vi "PlotMotionProfile.vi"(1 "Trajectory Points":T3[](array[typedef]) {"Time (ms)" items=["TrajectoryDuration_0ms"=0, "TrajectoryDuration_5ms"=5, "TrajectoryDuration_10ms"=10, "TrajectoryDuration_20ms"=20, "TrajectoryDuration_30ms"=30, "TrajectoryDuration_40ms"=40, "TrajectoryDuration_50ms"=50, "TrajectoryDuration_100ms"=100]}) -> (0 "MotionProfileGraph":T2 {"Trajectory Point Interval (ms)" items=["TrajectoryDuration_0ms"=0, "TrajectoryDuration_5ms"=5, "TrajectoryDuration_10ms"=10, "TrajectoryDuration_20ms"=20, "TrajectoryDuration_30ms"=30, "TrajectoryDuration_40ms"=40, "TrajectoryDuration_50ms"=50, "TrajectoryDuration_100ms"=100]})   [LabVIEW 2018, in "ArgosLib.lvlib"]
uses:
  ArgosLib.lvlib
  TypeDefs/TrajectoryPoint.ctl
  <vilib>/Rock Robotics/WPI/ThirdParty/Phoenix-LabVIEW/Motor Controller/Controls/CTRE_Phoenix_MotorControl_TrajectoryPointTimeDur.ctl
panel:
  # "Wire this output to a waveform graph.\nPlot 0 is position\nPlot 1 is velocity\nPlot 2 is acceleration"
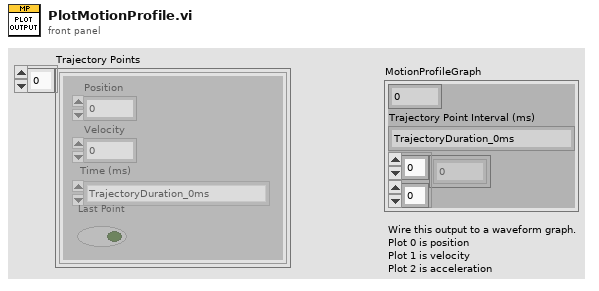
[diagram p1: front panel]
types:
  T1 = typedef "CTRE_Phoenix_MotorControl_TrajectoryPointTimeDur.ctl" = i32
  T2 = cluster{dbl, "Trajectory Point Interval (ms)":T1, dbl[][]}
  T3 = typedef "ArgosLib.lvlib/TrajectoryPoint.ctl" = cluster{"Position ":dbl, "Velocity ":dbl, "Time (ms)":T1, "Last Point":bool}
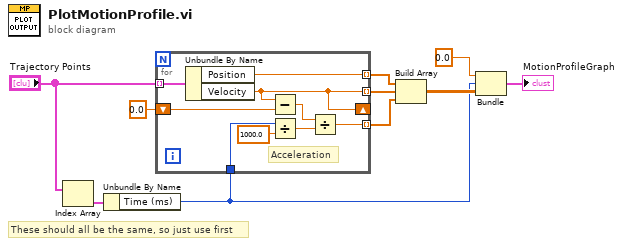
[diagram p0: block diagram]
diagram:
  # "These should all be the same, so just use first"
  n1 = Index Array(array="Trajectory Points") -> (element=w2:T3)  [unwired: 1 in]
  n2 = Unbundle By Name(w2) -> ("Time (ms)"=w1:T1)
  n3 = for {
    tunnel: "Trajectory Points" -> [w19] mode=indexing
    tunnel: [w18] -> w9 mode=indexing
    tunnel: [w17] -> w8 mode=indexing
    shift-right: [w17] -> _
    shift-left: 0.0 ("Velocity") -> [w16]
    tunnel: [w14] -> w5 mode=indexing
    tunnel: w1 -> [w13]
    # "Acceleration"
    n4 = Unbundle By Name(w19) -> ("Position"=w18:dbl, "Velocity"=w17:dbl)
    n5 = Subtract(x=w17, y=w16) -> (x-y=w15:dbl)
    n6 = Divide(x=w13, y=1000.0) -> (x/y=w11:dbl)
    n7 = Divide(x=w15, y=w11) -> (x/y=w14:dbl)
  }
  n8 = Build Array(w9, w8, w5) -> (w7:dbl[][])
  n9 = Bundle(0.0, "Time (ms)"=w1, w7) -> (→"MotionProfileGraph":cluster{dbl, "Time (ms)":T1, dbl[][]})  [unwired: 1 in]
